vi "Get TimerDRV.vi"(11 "FRTS Process in":refnum<class "FRTS Process.lvclass">) -> (2 "TimingDRV Engine.lvlib:TimerDRV.lvclass":refnum<class "TimerDRV.lvclass">, 3 "FRTS Process out":refnum<class "FRTS Process.lvclass">)   [LabVIEW 2019, in "TimingDRV Engine.lvlib" / "FRTS Process.lvclass"]
uses:
  FRTS Process.lvclass
  Parent Classes/TimerDRV Class/TimerDRV.lvclass
  FRTS Process.lvclass/FRTS Process.ctl
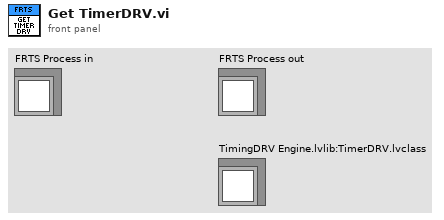
[diagram p1: front panel]
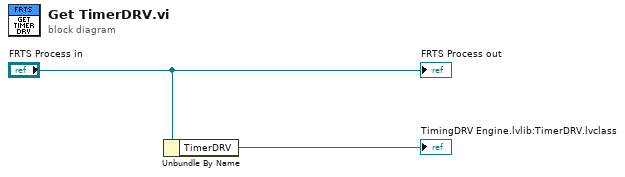
[diagram p0: block diagram]
diagram:
  n1 = Unbundle By Name("FRTS Process in") -> ("TimerDRV"=→"TimingDRV Engine.lvlib:TimerDRV.lvclass":refnum<class "TimerDRV.lvclass">)
  "FRTS Process out" <- "FRTS Process in"
